vi "Periodic Tasks.vi"(8 "error in":errorcluster) -> ()   [LabVIEW 2020]
doc: "This VI runs in parallel to other tasks. It can contain as many user-defined periodic loops as you need. These can carry out PID or other sorts of timed response."
uses:
  <vilib>/Rock Robotics/WPI/Compressor/WPI_CompressorFeedbackMode.ctl
  <vilib>/Rock Robotics/WPI/Utilities/WPI_GetSetVariantRefNum.vi
panel:
  out "Compressor Running":bool
  out "Enabled":bool
  in  "Disable Compressor":bool
  out "Pressure 0 (psi)":dbl(slide) scale=0.0..120.0
  in  "Enable Compressor Hybrid":bool
  in  "Min Pressure (PSI)":dbl(slide)=100.0 scale=0.0..120.0
  in  "Max Pressure (PSI)":dbl(slide)=120.0 scale=0.0..120.0
  # "Adjust the minimum and maximum pressure for\ncompressor control using the analog sensor.\n\nClick enable to enable compressor control\nwith the digital sensor and analog sensor.\n\nClick disable to stop the compressor regardless of\npressure."
  # "Compressor status"
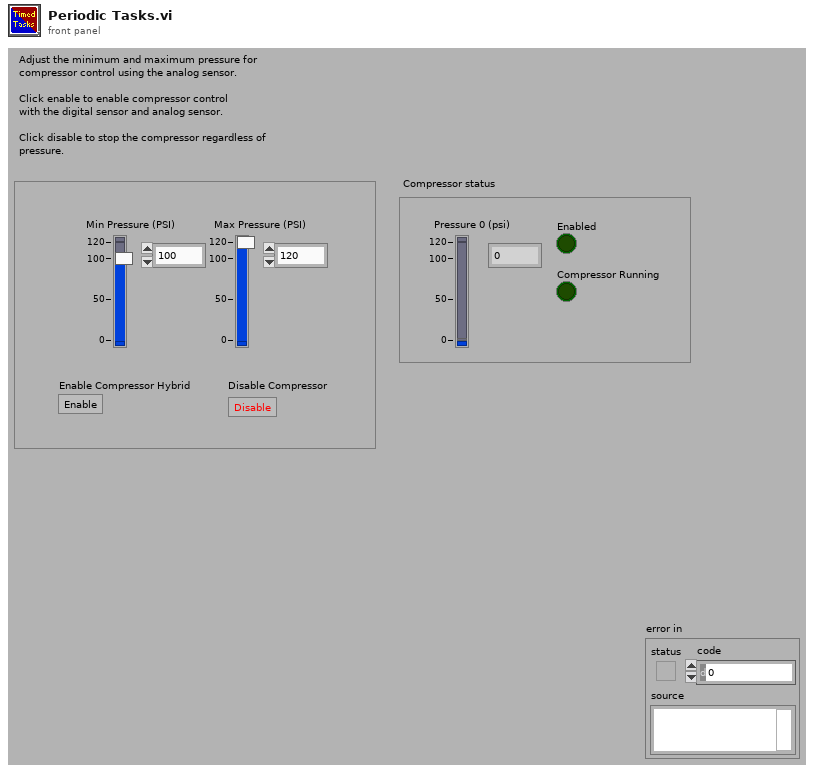
[diagram p1: front panel]
types:
  T1 = typedef "WPI_JoystickDevRef.ctl" = cluster{"Device":T2}
  T2 = typedef "WPI_JoystickDeviceEnum.ctl" = enum16{"USB 0", "USB 1", "USB 2", "USB 3", "USB 4", "USB 5"}
  T3 = typedef "WPI_RobotDriveDevRef.ctl" = cluster{"DevStatus":errorcluster, "Motors[]":T4[], "Square Inputs":bool, "Max Output":dbl}
  T4 = typedef "WPI_MotorControlDeviceRef.ctl" = cluster{"DeviceStatus":errorcluster, "Type":T5, "PWM":cluster{"PWM Channel":T6, "DeadBand":T7}, "CAN":cluster{"Device Number":u8, "SetOutput VI Ref":variant, "GetOutput VI Ref":variant, "Enable VI Ref":variant, "Disable VI Ref":variant, "Data":variant}, "Invert":bool, "DIO PWM":cluster{"PWM \"Enable\" Channel":T6, "DIOChannel":T8, "PWM Rate":dbl}}
  T5 = typedef "WPI_MotorControlType.ctl" = enum16{"PWM", "CAN", "DIO PWM"}
  T6 = typedef "FPGA_DIOPWMChannel.ctl" = enum8{"PWM 0", "PWM 1", "PWM 2", "PWM 3", "PWM 4", "PWM 5", "PWM 6", "PWM 7", "PWM 8", "PWM 9", "PWM MXP 0", "PWM MXP 1", "PWM MXP 2", "PWM MXP 3", "PWM MXP 4", "PWM MXP 5", "PWM MXP 6", "PWM MXP 7", "PWM MXP 8", "PWM MXP 9", "Invalid"}
  T7 = typedef "WPI_PWMDeadband.ctl" = cluster{"Name":string, "maxPositivePwm":i32, "minPositivePwm":i32, "centerPwm":i32, "maxNegativePwm":i32, "minNegativePwm":i32, "angularRange":u16}
  T8 = typedef "FPGA_DIOChannel.ctl" = enum8{"DIO 0", "DIO 1", "DIO 2", "DIO 3", "DIO 4", "DIO 5", "DIO 6", "DIO 7", "DIO 8", "DIO 9", "DIO MXP 0", "DIO MXP 1", "DIO MXP 2", "DIO MXP 3", "DIO MXP 4", "DIO MXP 5", "DIO MXP 6", "DIO MXP 7", "DIO MXP 8", "DIO MXP 9", "DIO MXP 10", "DIO MXP 11", "DIO MXP 12", "DIO MXP 13", "DIO MXP 14", "DIO MXP 15", "SPI Port CS1", "SPI Port CS2", "SPI Port CS3", "SPI Port MISO", "SPI Port MOSI", "Invalid"}
  T9 = cluster{"JoystickDevRef":T1, "RobotDriveDevRef":T3}
  T10 = typedef "WPI_CompressorDevRef.ctl" = cluster{"DevStatus":errorcluster, "Pneumatics Control Module":u8}
  T11 = typedef "WPI_CompressorFeedbackMode.ctl" = enum16{"Analog Only", "Digital Only", "Hybrid"}
  T12 = cluster{"Feedback Sensor":T11, "Max Pressure (PSI)":dbl, "Min Pressure (PSI)":dbl}
  T13 = cluster{"Pressure 0 (psi)":dbl, "Pressure 1 (psi)":dbl}
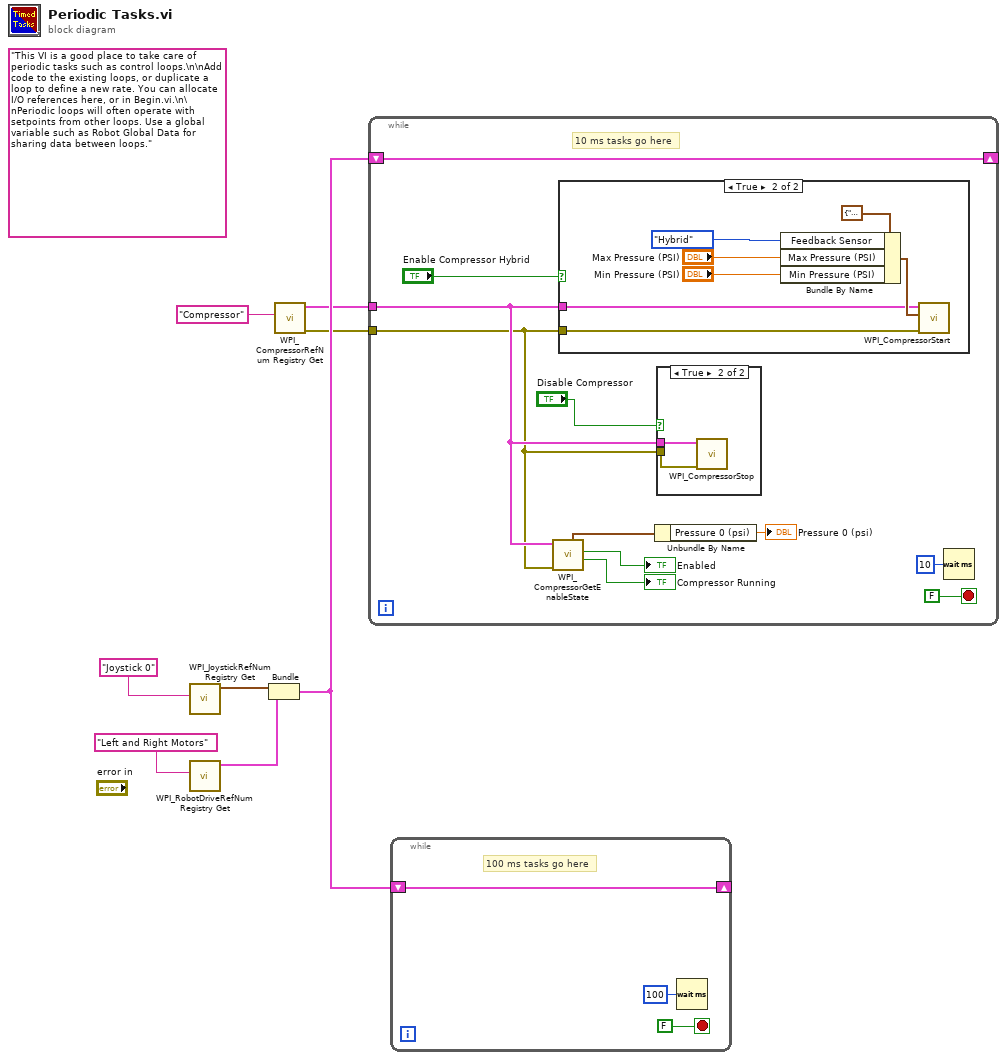
[diagram p0: block diagram]
diagram:
  (unwired) "This VI is a good place to take care of periodic tasks such as control loops.\n\nAdd code to the existing loops, or duplicate a loop to define a new rate. You can allocate I/O references here, or in Begin.vi.\n\nPeriodic loops will often operate with setpoints from other loops. Use a global variable such as Robot Global Data for sharing data between loops."
  n1 = call <vilib>:"WPI_JoystickRefNum Registry Get.vi"("refnum name"="Joystick 0") -> ("JoystickDevRef"=w6:T1)  [unwired: 1 in, 9 out]
  n2 = call <vilib>:"WPI_RobotDriveRefNum Registry Get.vi"("refnum name"="Left and Right Motors") -> ("RobotDriveDevRef"=w5:T3)  [unwired: 1 in, 9 out]
  n3 = Bundle("JoystickDevRef"=w6, "RobotDriveDevRef"=w5) -> (w4:T9)  [unwired: 1 out]
  n4 = call <vilib>:"WPI_CompressorRefNum Registry Get.vi"("refnum name"="Compressor") -> ("error out"=w1:errorcluster, "CompressorDevRef"=w2:T10)  [unwired: 9 in]
  n5 = while {
    shift-right: [w17] -> _
    shift-left: w4 -> [w17]
    tunnel: w2 -> [w10]
    tunnel: w1 -> [w9]
    stop <- FALSE stop-if-true
    # "10 ms tasks go here"
    n6 = call <vilib>:"WPI_CompressorGetEnableState.vi"("error in (no error)"=w9, "CompressorDevRef"=w10) -> ("Compressor Running"=→"Compressor Running":bool, "Enabled"=→"Enabled":bool, "Pressure Sensors"=w15:T13)  [unwired: 3 in, 4 out]
    n7 = case shown="True" "Enable Compressor Hybrid" {
      tunnel: w10 -> [_ w25]
      tunnel: w9 -> [_ w24]
      frame False {
      }
      frame True {
        n8 = Bundle By Name(cluster=T12 {"Feedback Sensor"=enum."Digital Only", "Max Pressure (PSI)"=0.0, "Min Pressure (PSI)"=0.0} ("Feedback Configuration"), "Feedback Sensor"=WPI_CompressorFeedbackMode."Hybrid", "Max Pressure (PSI)"="Max Pressure (PSI)", "Min Pressure (PSI)"="Min Pressure (PSI)") -> (w26:T12)
        n9 = call <vilib>:"WPI_CompressorStart.vi"("error in (no error)"=w24, "Feedback Configuration"=w26, "CompressorDevRef"=w25) -> ()  [unwired: 7 in, 2 out]
      }
    }
    n10 = Unbundle By Name(w15) -> ("Pressure 0 (psi)"=→"Pressure 0 (psi)":dbl)
    n11 = case shown="True" "Disable Compressor" {
      tunnel: w9 -> [_ w21]
      tunnel: w10 -> [_ w20]
      frame False {
      }
      frame True {
        n12 = call <vilib>:"WPI_CompressorStop.vi"("error in (no error)"=w21, "CompressorDevRef"=w20) -> ()  [unwired: 8 in, 2 out]
      }
    }
    n13 = Wait (ms)(milliseconds to wait=u32 10) -> ()  [unwired: 1 out]
  }
  n14 = while {
    shift-right: [w29] -> _
    shift-left: w4 -> [w29]
    stop <- FALSE stop-if-true
    # "100 ms tasks go here"
    n15 = Wait (ms)(milliseconds to wait=u32 100) -> ()  [unwired: 1 out]
  }
